vi "audio-stim-play.vi"(11 "Stimulus List":dbl[][](array[numeric])=[[0.0, 3.0, 0.2, 1.0, 500.0], [1.0, 3.0, 0.2, 1.0, 500.0], [2.0, 3.0, 0.2, 1.0, 500.0], [3.0, 3.0, 0.2, 1.0, 1000.0], [4.0, 3.0, 0.2, 1.0, 500.0], [5.0, 3.0, 0.2, 1.0, 500.0], [6.0, 3.0, 0.2, 1.0, 1000.0], [7.0, 3.0, 0.2, 1.0, 1000.0], [8.0, 3.0, 0.2, 1.0, 1000.0], [9.0, 3.0, 0.2, 1.0, 500.0], [10.0, 3.0, 0.2, 1.0, 500.0], [11.0, 3.0, 0.2, 1.0, 1000.0], [12.0, 3.0, 0.2, 1.0, 1000.0], [13.0, 3.0, 0.2, 1.0, 1000.0], [14.0, 3.0, 0.2, 1.0, 1000.0], [15.0, 3.0, 0.2, 1.0, 1000.0], [16.0, 3.0, 0.2, 1.0, 500.0], [17.0, 3.0, 0.2, 1.0, 500.0], [18.0, 3.0, 0.2, 1.0, 500.0], [19.0, 3.0, 0.2, 1.0, 1000.0]]) -> (3 "Playing":bool=TRUE caption="Playing stimulus")   [LabVIEW 2013]
uses:
  <vilib>/DAQmx/write.llb/DAQmx Write (Digital U16 1Chan 1Samp).vi
  <vilib>/DAQmx/write.llb/DAQmx Write (Analog Wfm 1Chan NSamp).vi
  <vilib>/DAQmx/create/channels.llb/DAQmx Create Channel (AO-Voltage-Basic).vi
  <vilib>/DAQmx/create/channels.llb/DAQmx Create Channel (DO-Digital Output).vi
  <vilib>/DAQmx/miscellaneous.llb/DAQmx Fill In Error Info.vi
  <vilib>/DAQmx/configure/timing.llb/DAQmx Timing (Use Waveform).vi
panel:
  out "Log File Path":path
  in  "Play Interval Jitter (s)":dbl=0.5
  in  "Play Interval (s)":dbl=1.0
  out "error out":errorcluster
  in  "DO Ports":tag="Dev1/port0:1" caption="DO Ports\n(\"browse\" and select two 8 bit ports)"
  in  "Sound AO Channel":tag="Dev1/ao0"
  out "Curr Param":dbl[](array[numeric])=[0.0, 3.0, 0.2, 1.0, 500.0] caption="Current (or Cued) Trial Parameters"
  in  "Sampling Rate":dbl=100000.0
  in  "stop":bool
  in  "Play":bool
  out "Current (or Cued) Waveform":waveform(dbl)(graph)={"t0"=timestamp(0 s since 1904-01-01), "dt"=1e-05, "Y"=array[19999 elements]}
  out "Waiting":bool=TRUE
  in  "Current (or Cued) Trial":i32(slide) min=0 max=20 scale=0.0..20.0
  # "Stim#, Stim Type, Duration, Amplitude, Param 1, Param 2, Param 3, Param 4"
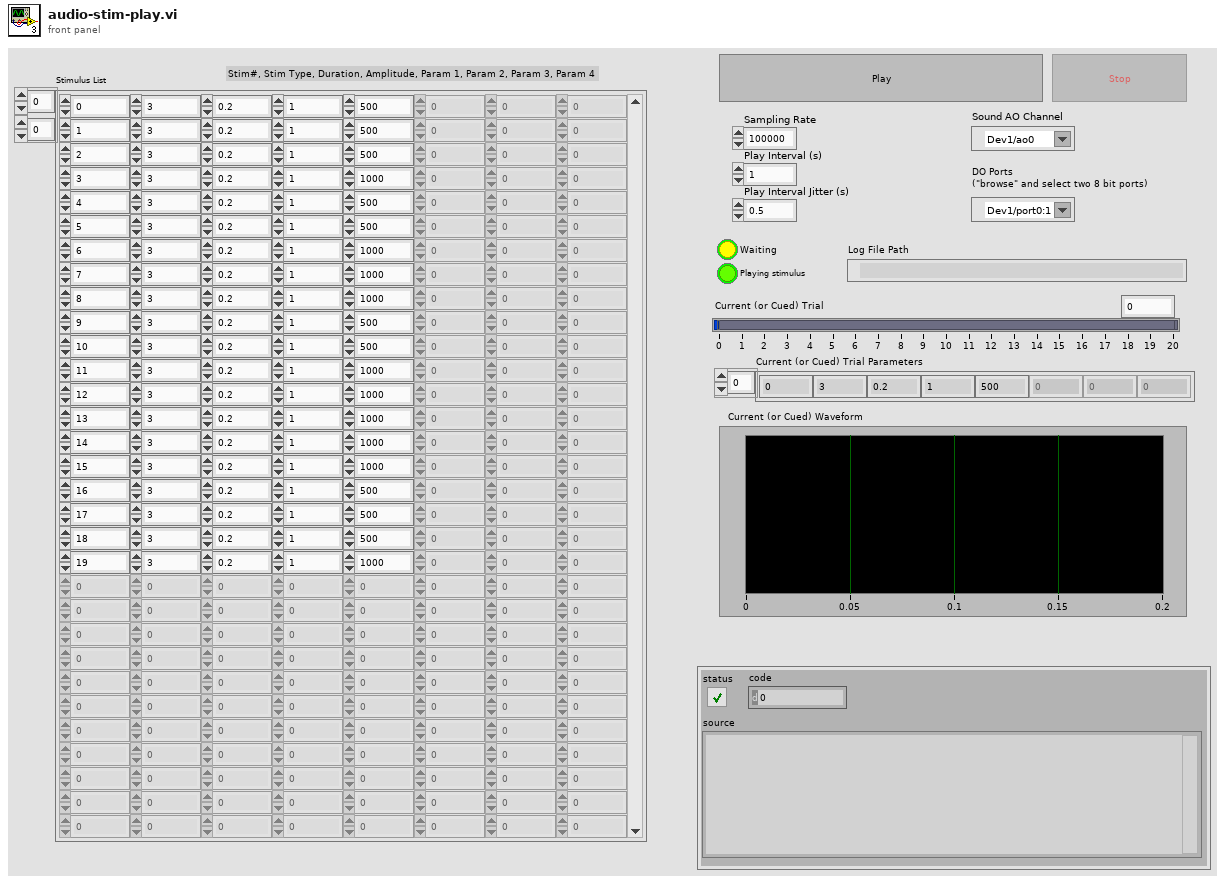
[diagram p1: front panel]
types:
  T1 = cluster{"Sampling Rate":dbl, "Value 3":dbl, dbl, "Value 2":dbl}
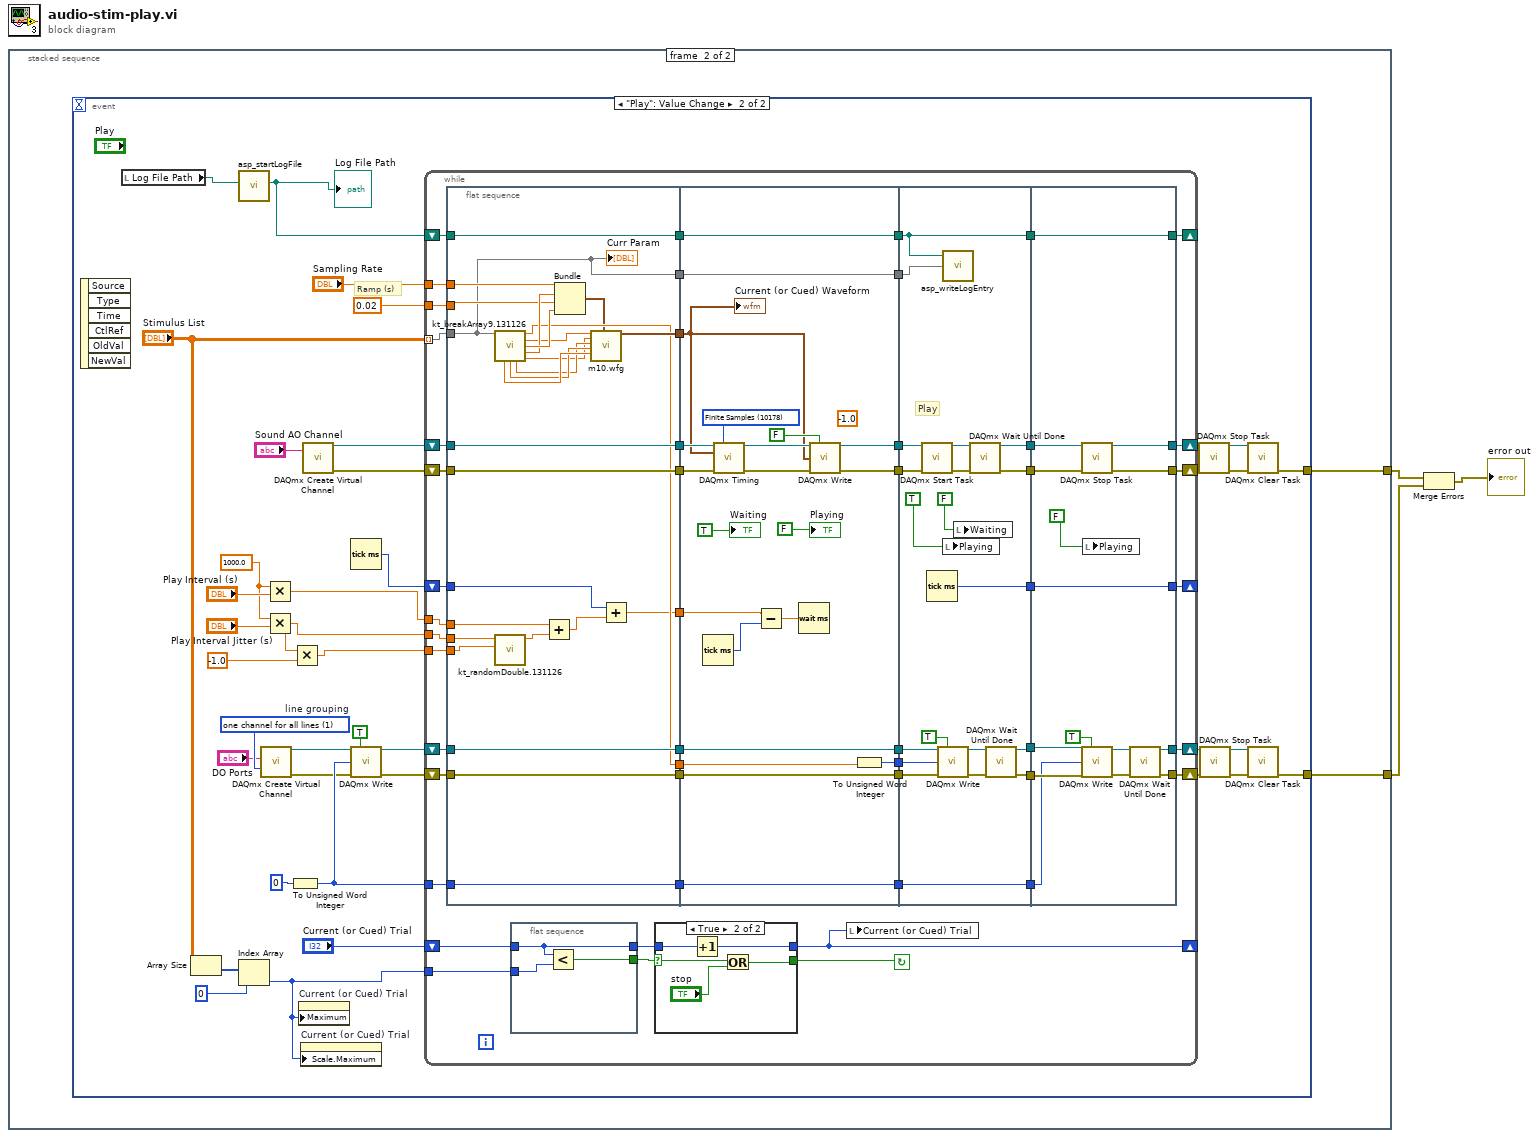
[diagram p0: block diagram]
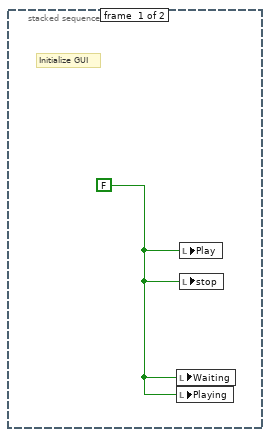
[diagram p2: hidden frame]
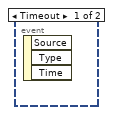
[diagram p3: hidden frame]
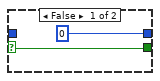
[diagram p4: hidden frame]
diagram:
  n1 = stacked-sequence {
    tunnel: [_ w6] -> w3
    tunnel: [_ w5] -> w2
    frame #0 {
      w4 = FALSE ("Play")
      # "Initialize GUI"
      n2 = local write "Waiting"(w4) -> ()
      n3 = local write "Playing"(w4) -> ()
      n4 = local write "Play"(w4) -> ()
      n5 = local write "stop"(w4) -> ()
    }
    frame #1 {
      n6 = event shown="[1] \"Play\": Value Change" {
        selector: _ -> [_ _]
        dyn-events: _ -> [_ _]
        timeout: _ -> [_ _]
        tunnel: [_ w21] -> w6
        tunnel: [_ w20] -> w5
        event Timeout {
          n7 = event-data() -> ()  [unwired: 1 in, 3 out]
        }
        event "Play": Value Change {
          w13 = 1000.0 ("y")
          w42 = 1 items=["one channel for each line", "one channel for all lines"]  # line grouping
          # "Ramp (s)"
          n8 = event-data() -> ()  [unwired: 1 in, 6 out]
          n9 = local read "Log File Path"() -> (w8:path)
          n10 = Array Size(array="Stimulus List") -> (size(s)=w40:i32[])
          n11 = call "asp_startLogFile.vi"("Path In"=w8) -> ("Path"=w7:path)  [unwired: 5 in, 1 out]
          "Log File Path" <- w7
          n12 = Index Array(array=w40, index=0) -> (element=w24:i32)
          n13 = call-poly <vilib>:"DAQmx Create Virtual Channel.vi"("lines"="DO Ports", "line grouping"=w42) -> ("task out"=w18:refnum<k21>, "error out"=w17:errorcluster)  [unwired: 12 in]
          n14 = Multiply(x=w13, y="Play Interval (s)") -> (x*y=w12:dbl)
          n15 = Multiply(x=w13, y="Play Interval Jitter (s)") -> (x*y=w10:dbl)
          n16 = To Unsigned Word Integer(number=u16 0 ("data")) -> (unsigned 16bit integer=w25:u16)
          n17 = Multiply(x=w10, y=-1.0) -> (x*y=w11:dbl)
          n18 = property on="Current (or Cued) Trial" class="Slide (strict)"("Maximum"=w24) -> ()  [unwired: 2 in, 2 out]
          n19 = property on="Current (or Cued) Trial" class="Slide (strict)"("Scale.Maximum"=w24) -> ()  [unwired: 2 in, 2 out]
          n20 = call-poly <vilib>:"DAQmx Create Virtual Channel.vi"("physical channels"="Sound AO Channel") -> ("task out"=w23:refnum<k21>, "error out"=w22:errorcluster)  [unwired: 13 in]
          n21 = Tick Count (ms)() -> (millisecond timer value=w9:u32)
          n22 = call-poly <vilib>:"DAQmx Write.vi"("task/channels in"=w18, "auto start"=TRUE, "data"=w25, "error in"=w17) -> ("task out"=w29:refnum<k21>, "error out"=w28:errorcluster)  [unwired: 9 in, 1 out]
          n23 = while {
            tunnel: "Stimulus List" -> [w63] mode=indexing
            tunnel: "Sampling Rate" -> [w62]
            tunnel: 0.02 -> [w61]
            shift-right: [w93] -> w34
            shift-left: w23 -> [w91]
            shift-right: [w92] -> w33
            shift-left: w22 -> [w90]
            shift-right: [w80] -> w38
            shift-left: w29 -> [w89]
            shift-right: [w79] -> w37
            shift-left: w28 -> [w71]
            shift-right: [w74] -> _
            shift-left: "Current (or Cued) Trial" -> [w83]
            tunnel: w24 -> [w82]
            tunnel: w25 -> [w77]
            shift-right: [w58] -> _
            shift-left: w9 -> [w57]
            tunnel: w12 -> [w53]
            tunnel: w11 -> [w54]
            tunnel: w10 -> [w55]
            shift-right: [w46] -> _
            shift-left: w7 -> [w52]
            stop <- w72 continue-if-true
            n24 = flat-sequence {
              tunnel: w71 -> [w127]
              tunnel: w77 -> [w128]
              tunnel: w89 -> [w129]
              tunnel: w90 -> [w130]
              tunnel: w91 -> [w131]
              tunnel: [w131] -> w69
              tunnel: [w130] -> w68
              tunnel: [w129] -> w67
              tunnel: [w128] -> w66
              tunnel: [w127] -> w65
              tunnel: [w119] -> w64
              tunnel: w63 -> [w106]
              tunnel: w62 -> [w118]
              tunnel: w61 -> [w117]
              tunnel: [w116] -> w60
              tunnel: w57 -> [w114]
              tunnel: [w113] -> w56
              tunnel: w55 -> [w112]
              tunnel: w54 -> [w111]
              tunnel: w53 -> [w108]
              tunnel: w52 -> [w107]
              tunnel: [w107] -> w51
              tunnel: [w106] -> w50
              tunnel: [w142] -> w95
              tunnel: [w141] -> w94
              tunnel: [w151] -> w88
              tunnel: [w150] -> w81
              tunnel: [w149] -> w78
              tunnel: [w139] -> w70
              tunnel: w69 -> [w148]
              tunnel: w68 -> [w147]
              tunnel: w67 -> [w151]
              tunnel: w66 -> [w149]
              tunnel: w65 -> [w139]
              tunnel: w64 -> [w138]
              tunnel: w60 -> [w137]
              tunnel: w56 -> [w134]
              tunnel: w51 -> [w132]
              tunnel: w50 -> [w133]
              tunnel: [w133] -> w49
              tunnel: [w132] -> w48
              tunnel: w95 -> [w162]
              tunnel: w94 -> [w161]
              tunnel: w88 -> [w170]
              tunnel: [w164] -> w87
              tunnel: [w163] -> w86
              tunnel: [w167] -> w85
              tunnel: [w166] -> w84
              tunnel: w81 -> [w171]
              tunnel: w78 -> [w165]
              tunnel: [w165] -> w76
              tunnel: w70 -> [w156]
              tunnel: [w155] -> w59
              tunnel: w49 -> [w154]
              tunnel: w48 -> [w153]
              tunnel: [w153] -> w47
              tunnel: [w175] -> w92
              tunnel: [w176] -> w93
              tunnel: w87 -> [w178]
              tunnel: w86 -> [w177]
              tunnel: w85 -> [w186]
              tunnel: w84 -> [w185]
              tunnel: [w181] -> w80
              tunnel: [w180] -> w79
              tunnel: w76 -> [w179]
              tunnel: w59 -> [w174]
              tunnel: [w174] -> w58
              tunnel: w47 -> [w173]
              tunnel: [w173] -> w46
              frame #0 {
                n25 = call "kt_breakArray9.131126.vi"("Current (or Cued Trial Parameters)"=w106) -> ("Value 0"=w116:dbl, "Value 1"=w120:dbl, "Value 2"=w122:dbl, "Value 3"=w121:dbl, "Value 7"=w126:dbl, "Value 6"=w125:dbl, "Value 5"=w124:dbl, "Value 4"=w123:dbl)  [unwired: 6 in, 1 out]
                n26 = call "kt_randomDouble.131126.vi"("Min"=w111, "Max"=w112) -> ("Random"=w109:dbl)  [unwired: 9 in]
                n27 = Add(x=w108, y=w109) -> (x+y=w110:dbl)
                n28 = Bundle("Sampling Rate"=w118, "Value 3"=w121, w117, "Value 2"=w122) -> (w115:T1)  [unwired: 1 in]
                n29 = call "m10.wfg.vi"("Stimulus Type"=w120, "Param 0"=w123, "Param 1"=w124, "Param 2"=w125, "Param 3"=w126, "Waveform Properties"=w115) -> ("Waveform Out"=w119:waveform(dbl))  [unwired: 12 in, 1 out]
                n30 = Add(x=w114, y=w110) -> (x+y=w113:dbl)
                "Curr Param" <- w106
              }
              frame #1 {
                (unwired) -1.0 ("timeout")
                w146 = 10178 items=["Finite Samples"=10178, "Continuous Samples"=10123, "Hardware Timed Single Point"=12522] ("sample mode")
                n31 = Tick Count (ms)() -> (millisecond timer value=w135:u32)
                n32 = call-poly <vilib>:"DAQmx Timing.vi"("task/channels in"=w148, "sample mode"=w146, "waveform"=w138, "error in"=w147) -> ("task out"=w145:refnum<k21>, "error out"=w144:errorcluster)  [unwired: 10 in]
                n33 = Subtract(x=w134, y=w135) -> (x-y=w136:dbl)
                n34 = Wait (ms)(milliseconds to wait=w136) -> ()  [unwired: 1 out]
                n35 = call-poly <vilib>:"DAQmx Write.vi"("task/channels in"=w145, "auto start"=FALSE, "data"=w138, "error in"=w144) -> ("task out"=w142:refnum<k21>, "error out"=w141:errorcluster)  [unwired: 9 in, 1 out]
                n36 = To Unsigned Word Integer(number=w137) -> (unsigned 16bit integer=w150:u16)
                "Waiting" <- TRUE ("Playing Stimulus")
                "Playing" <- FALSE ("Playing Stimulus")
                "Current (or Cued) Waveform" <- w138
              }
              frame #2 {
                # "Play"
                n37 = call <vilib>:"DAQmx Start Task.vi"("task/channels in"=w162, "error in"=w161) -> ("task out"=w160:refnum<k21>, "error out"=w159:errorcluster)  [unwired: 12 in]
                n38 = Tick Count (ms)() -> (millisecond timer value=w155:u32)
                n39 = call-poly <vilib>:"DAQmx Write.vi"("task/channels in"=w170, "auto start"=TRUE, "data"=w171, "error in"=w156) -> ("task out"=w169:refnum<k21>, "error out"=w168:errorcluster)  [unwired: 9 in, 1 out]
                n40 = call "asp_writeLogEntry.vi"("Path In"=w153, "Curr Param"=w154) -> ()  [unwired: 4 in, 1 out]
                n41 = local write "Playing"(TRUE ("Playing Stimulus")) -> ()
                n42 = local write "Waiting"(FALSE ("Playing Stimulus")) -> ()
                n43 = call <vilib>:"DAQmx Wait Until Done.vi"("task/channels in"=w160, "error in"=w159) -> ("task out"=w164:refnum<k21>, "error out"=w163:errorcluster)  [unwired: 12 in]
                n44 = call <vilib>:"DAQmx Wait Until Done.vi"("task/channels in"=w169, "error in"=w168) -> ("task out"=w167:refnum<k21>, "error out"=w166:errorcluster)  [unwired: 12 in]
              }
              frame #3 {
                n45 = call <vilib>:"DAQmx Stop Task.vi"("task/channels in"=w178, "error in"=w177) -> ("task out"=w176:refnum<k21>, "error out"=w175:errorcluster)  [unwired: 12 in]
                n46 = call-poly <vilib>:"DAQmx Write.vi"("task/channels in"=w186, "auto start"=TRUE, "data"=w179, "error in"=w185) -> ("task out"=w183:refnum<k21>, "error out"=w182:errorcluster)  [unwired: 9 in, 1 out]
                n47 = local write "Playing"(FALSE ("Playing Stimulus")) -> ()
                n48 = call <vilib>:"DAQmx Wait Until Done.vi"("task/channels in"=w183, "error in"=w182) -> ("task out"=w181:refnum<k21>, "error out"=w180:errorcluster)  [unwired: 12 in]
              }
            }
            n49 = flat-sequence {
              tunnel: w83 -> [w103]
              tunnel: w82 -> [w105]
              tunnel: [w104] -> w73
              tunnel: [w103] -> w75
              frame #0 {
                n50 = Less?(x=w103, y=w105) -> (x < y?=w104:bool)
              }
            }
            n51 = case shown="True" w73 {
              selector: w73 -> [w96 w99]
              tunnel: w75 -> [_ w102]
              tunnel: [0 w101] -> w74
              tunnel: [w96 w100] -> w72
              frame False {
              }
              frame True {
                n52 = Increment(x=w102) -> (x+1=w101:i32)
                n53 = Or(x=w99, y="stop") -> (x .or. y?=w100:bool)
              }
            }
            n54 = local write "Current (or Cued) Trial"(w74) -> ()
          }
          n55 = call <vilib>:"DAQmx Stop Task.vi"("task/channels in"=w34, "error in"=w33) -> ("task out"=w32:refnum<k21>, "error out"=w31:errorcluster)  [unwired: 12 in]
          n56 = call <vilib>:"DAQmx Stop Task.vi"("task/channels in"=w38, "error in"=w37) -> ("task out"=w36:refnum<k21>, "error out"=w35:errorcluster)  [unwired: 12 in]
          n57 = call <vilib>:"DAQmx Clear Task.vi"("task in"=w32, "error in"=w31) -> ("error out"=w21:errorcluster)  [unwired: 13 in]
          n58 = call <vilib>:"DAQmx Clear Task.vi"("task in"=w36, "error in"=w35) -> ("error out"=w20:errorcluster)  [unwired: 13 in]
        }
      }
    }
  }
  n59 = Merge Errors(w3, w2) -> (→"error out":errorcluster)
